vi "CLD 1 Elapsed Time Express Solution.vi"() -> ()   [LabVIEW 2019]
doc: "CLD exercise 1\n\nThis VI is a caller for the Express VI. This Express VI is reentrant, so care must be taken if more than one is used in a VI."
panel:
  out "Elapsed Time (s)":dbl
  out "Time Has Elapsed":bool
  in  "Auto Reset":bool=TRUE
  in  "Reset Button":bool
  in  "Stop VI":bool
  out "error out":errorcluster
  in  "error in (no error)":errorcluster
  in  "Time Target (s)":dbl=2.0
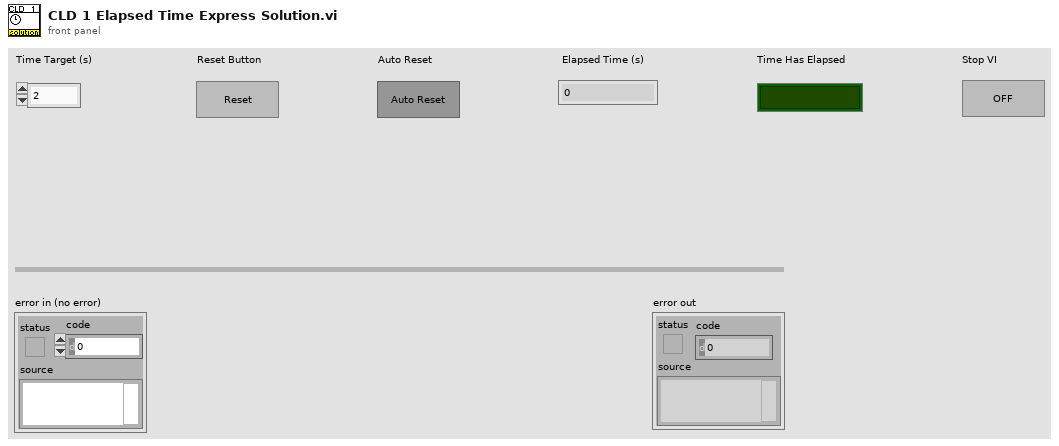
[diagram p1: front panel]
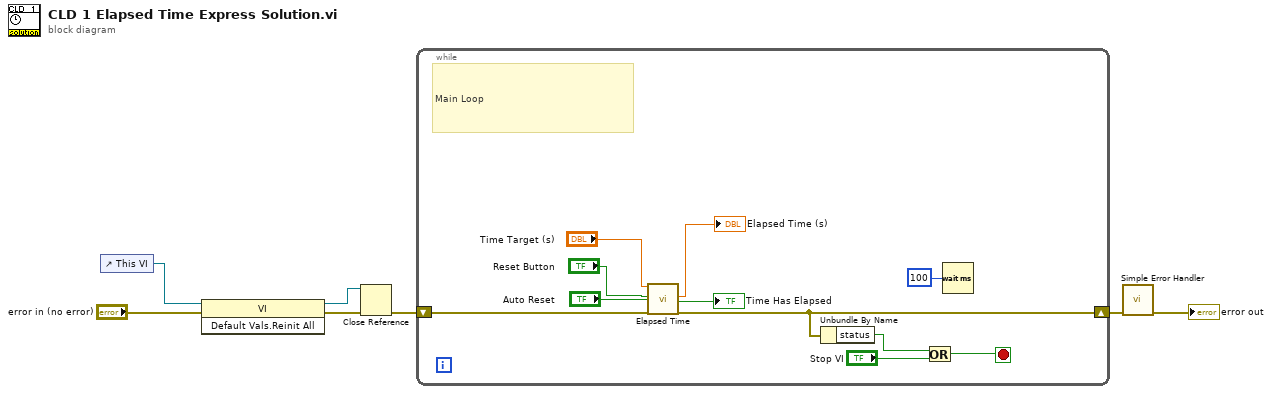
[diagram p0: block diagram]
diagram:
  n1 = control-ref of="This VI"() -> (w4:refnum<vi>)
  n2 = invoke class="VI" method="Default Vals.Reinit All"(reference=w4, error in="error in (no error)") -> (reference out=w2:refnum<vi>, error out=w5:errorcluster)  [unwired: 1 in, 1 out]
  n3 = Close Reference(reference=w2, error in (no error)=w5) -> (error out=w3:errorcluster)
  n4 = while {
    shift-right: [w12] -> w6
    shift-left: w3 -> [w16]
    stop <- w11 stop-if-true
    # "Main Loop"
    n5 = call "Elapsed Time"("Time Target (s)"="Time Target (s)", "Reset"="Reset Button", "Auto Reset"="Auto Reset", "error in (no error)"=w16) -> ("Elapsed Time (s)"=→"Elapsed Time (s)":dbl, "Time has Elapsed"=→"Time Has Elapsed":bool, "error out"=w12:errorcluster)  [unwired: 8 in, 5 out]
    n6 = Unbundle By Name(w12) -> ("status"=w10:bool)
    n7 = Or(x=w10, y="Stop VI") -> (x .or. y?=w11:bool)
    n8 = Wait (ms)(milliseconds to wait=u32 100) -> ()  [unwired: 1 out]
  }
  n9 = call <vilib>:"Simple Error Handler.vi"("error in (no error)"=w6) -> ("error out"=→"error out":errorcluster)  [unwired: 4 in, 4 out]
